vi "Noti_Reg.vi"(8 "error in (no error)":errorcluster, 11 "NotifyIcon in":refnum<class "NotifyIcon.lvclass">) -> (0 "error out":errorcluster, 3 "NotifyIcon out":refnum<class "NotifyIcon.lvclass">)   [LabVIEW 2016, in "NotifyIcon.lvclass"]
uses:
  NotifyIcon.lvclass
  System.Windows.Forms
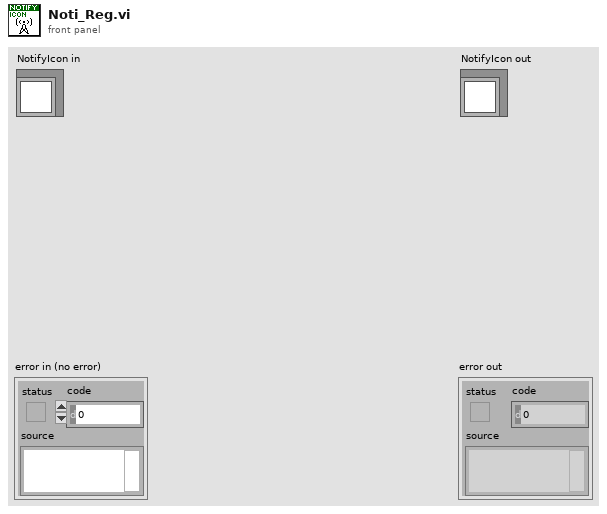
[diagram p1: front panel]
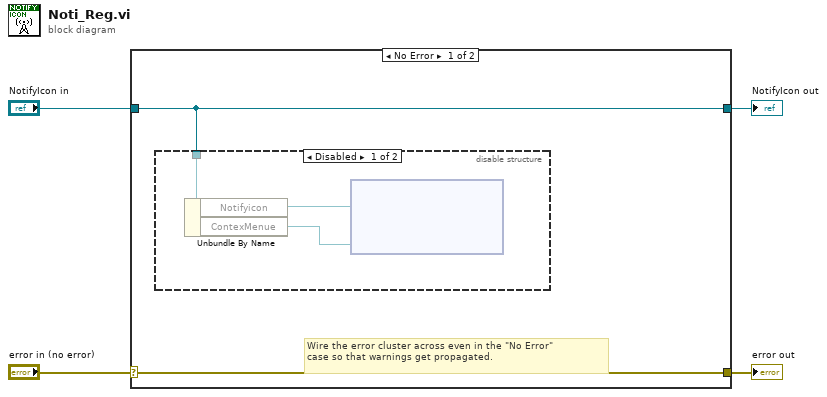
[diagram p0: block diagram]
diagram:
  n1 = case shown="No Error" "error in (no error)" {
    selector: "error in (no error)" -> [w6 w11]
    tunnel: [w6 w11] -> w3
    tunnel: [w5 w10] -> w1
    tunnel: "NotifyIcon in" -> [w5 w10]
    frame No Error {
      # "Wire the error cluster across even in the \"No Error\"\ncase so that warnings get propagated."
      n2 = disable-structure shown="Disabled" {
        disable-tunnel: w5 -> [w9 _]
        frame Disabled {
          n3 = Unbundle By Name(w9) -> ("Notifyicon"=w8:refnum<k24>, "ContexMenue"=w7:refnum<class "ContexMenue.lvclass">)
          n4 = node(w8, w7) -> ()  [unwired: 3 in, 2 out]
        }
        frame Enabled {
        }
      }
    }
    frame Error {
    }
  }
  "error out" <- w3
  "NotifyIcon out" <- w1
